vi "__ExtractHTMLSection.vi"(10 "Section to find":string, 11 "HTML String":string) -> (3 "Section":string)   [LabVIEW 2020, in "StashRoyale.lvclass"]
uses:
  StashRoyale.lvclass
panel:
  out "Array":i32[](array[numeric])
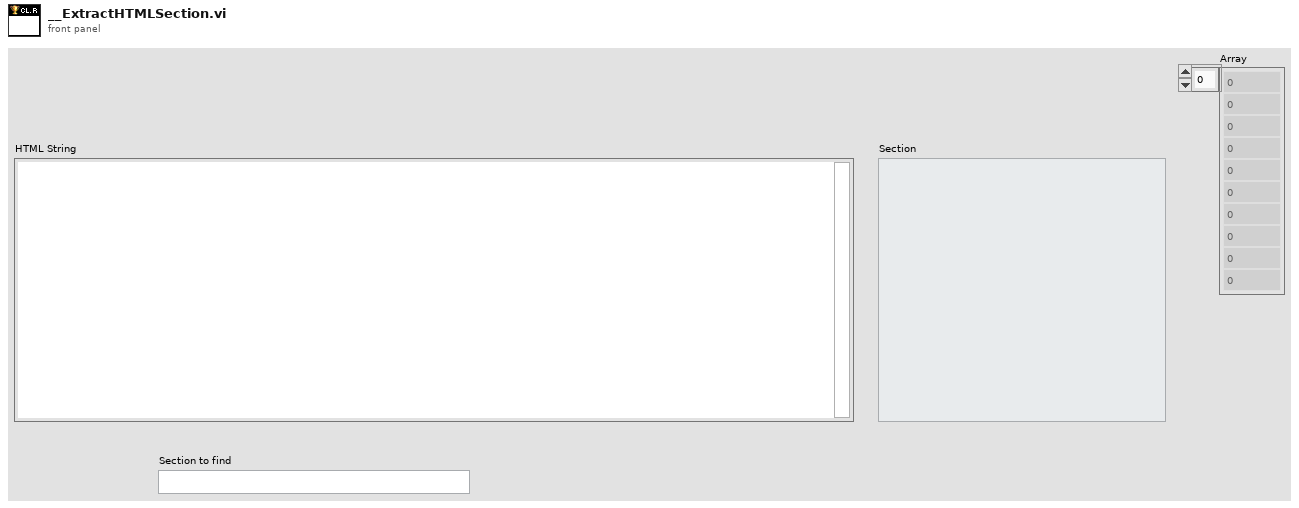
[diagram p1: front panel]
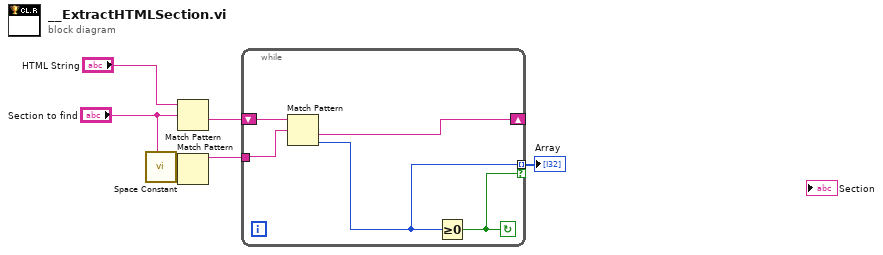
[diagram p0: block diagram]
diagram:
  n1 = call <vilib>:"Space Constant.vi"() -> ("String"=w4:string)
  n2 = Match Pattern(string="HTML String", regular expression="Section to find") -> (after substring=w3:string)  [unwired: 1 in, 3 out]
  n3 = Match Pattern(string="Section to find", regular expression=w4) -> (before substring=w2:string)  [unwired: 1 in, 3 out]
  n4 = while {
    shift-right: [w9] -> _
    shift-left: w3 -> [w11]
    tunnel: w2 -> [w10]
    tunnel: [w8] -> w1 mode=indexing if=w7
    stop <- w7 continue-if-true
    n5 = Match Pattern(string=w11, regular expression=w10) -> (after substring=w9:string, offset past match=w8:i32)  [unwired: 1 in, 2 out]
    n6 = Greater Or Equal To 0?(x=w8) -> (x >= 0?=w7:bool)
  }
  "Array" <- w1
